vi "Global.vi"() -> ()   [LabVIEW 2020]
panel:
  out "空载速度(°/s) 2":sgl format="%#_4g"
  in  "传感器码右":refnum<vi>
  in  "传感器码左":refnum<vi>
  out "右启用":i16
  out "左启用":i16
  out "右在位":i16
  out "左在位":i16
  out "跳转":i16
  out "右状态":i16
  out "左状态":i16
  out "设备状态":i16
  in  "计时开始":bool
  in  "计时复位":bool
  in  "IO_Stop":bool
  in  "上序状态":refnum<vi>
  out "右标定":dbl
  out "左标定":dbl
  out "扭矩":cluster{"工位一":dbl, "工位二":dbl}
  out "工位二扭矩偏移":cluster{"正向":dbl, "逆向":dbl}
  out "工位一扭矩偏移":cluster{"正向":dbl, "逆向":dbl}
  out "空载速度(°/s)":sgl
  in  "关闭client":bool
  in  "Result  右工位":refnum<vi>
  in  "合格数量":i32
  in  "生产数量":i32
  in  "试验项目":bool[](array[boolean])
  out "模式":u32
  in  "更换产品":refnum<vi>
  in  "提示信息":refnum<vi>
  in  "程序自动":refnum<vi>
  in  "报警图标":refnum<vi>
  in  "程序关闭":bool
  in  "Info":refnum<vi>
  in  "Result":refnum<vi>
  in  "批次":refnum<vi>
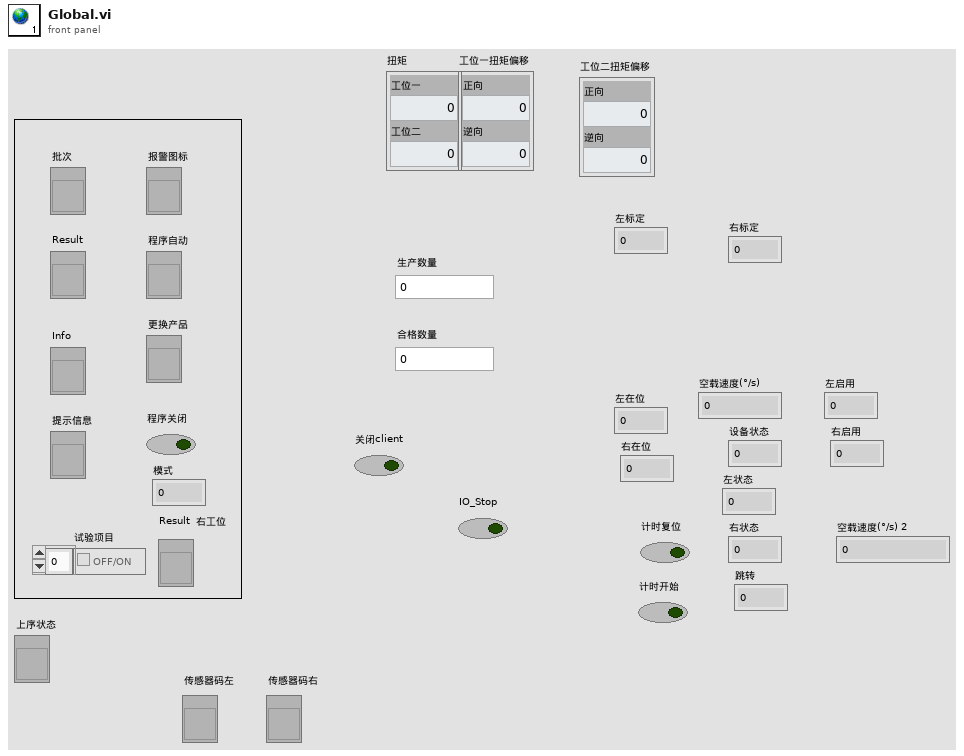
[diagram p1: front panel]
diagram:
